vi "Configure.vi"(8 "error in (no error)":errorcluster, 10 "Msg in":T1, 11 "FakePressureController in":refnum<class "Tapedrive_ESP301.lvclass">) -> (0 "error out":errorcluster, 1 "new command":string, 2 "Msg out":T1, 3 "FakePressureController out":refnum<class "Tapedrive_ESP301.lvclass">)   [LabVIEW 2011, in "Tapedrive_ESP301.lvclass"]
uses:
  Tapedrive_ESP301.lvclass
  DriverMsg.ctl
  Tapedrive_ESP301.lvclass/Tapedrive_ESP301.ctl
  OnOffTypeDef.ctl
  Direction.ctl
  BaseDriver/BaseDriver.lvclass
  Newport ESP301.lvlib
panel:
  out "Command":string
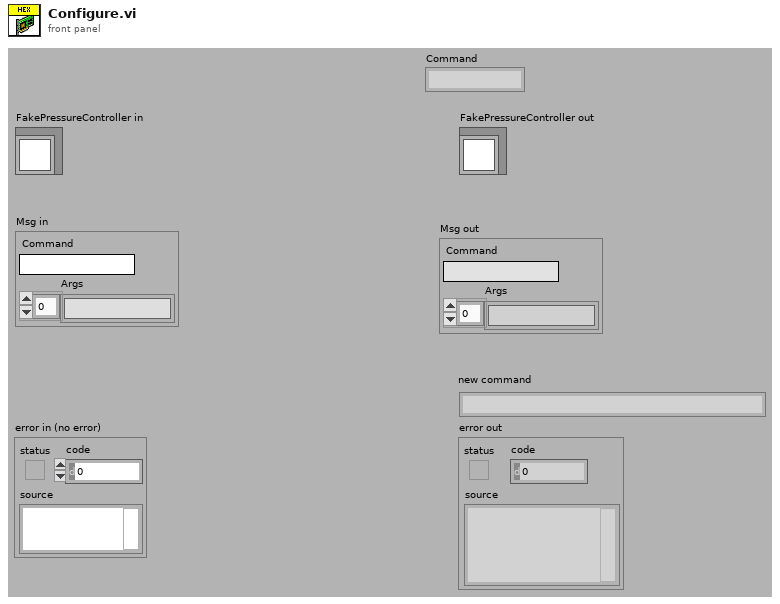
[diagram p1: front panel]
types:
  T1 = typedef "DriverMsg.ctl" = cluster{"Command":string, "Args":string[]}
  T2 = typedef "OnOffTypeDef.ctl" = enum16{"off", "on"}
  T3 = typedef "Direction.ctl" = enum16{"Forward", "Backward", "Undefined"}
  T4 = enum16{"Trapezoidal Mode", "S-curve Mode", "Jog Mode", "Slave to master's desired position (trajectory)", "Slave to master's actual position (feedback)", "Slave to master's actual velocity for jogging"}
  T5 = typedef "Tapedrive_ESP301.lvclass/settingsCluster_TapeDrive_TypDef.ctl" = cluster{"devport":string, "tapepos":cluster{"Value":dbl, "Min":dbl, "Max":dbl, "StepSize":dbl, "Tolerance":dbl, "ValueActual":dbl}, "status":enum16{"Not referenced", "Homing", "Moving", "Ready"}, "inmotion":T2, "forwardaxis":i16, "backwardaxis":i16, "encoderaxis":i16, "Velocity":cluster{"Axis 1":cluster{"Value":dbl, "Min":dbl, "Max":dbl, "StepSize":dbl, "Tolerance":dbl, "ValueActual":dbl}, "Axis 2":cluster{"Value":dbl, "Min":dbl, "Max":dbl, "StepSize":dbl, "Tolerance":dbl, "ValueActual":dbl}}, "Acceleration":cluster{"Axis 1":cluster{"Value":dbl, "Min":dbl, "Max":dbl, "StepSize":dbl, "Tolerance":dbl, "ValueActual":dbl}, "Axis 2":cluster{"Value":dbl, "Min":dbl, "Max":dbl, "StepSize":dbl, "Tolerance":dbl, "ValueActual":dbl}}, "Decceleration":cluster{"Axis 1":cluster{"Value":dbl, "Min":dbl, "Max":dbl, "StepSize":dbl, "Tolerance":dbl, "ValueActual":dbl}, "Axis 2":cluster{"Value":dbl, "Min":dbl, "Max":dbl, "StepSize":dbl, "Tolerance":dbl, "ValueActual":dbl}}, "MaxAcceleration":cluster{"Axis 1":cluster{"Value":dbl, "Min":dbl, "Max":dbl, "StepSize":dbl, "Tolerance":dbl, "ValueActual":dbl}, "Axis 2":cluster{"Value":dbl, "Min":dbl, "Max":dbl, "StepSize":dbl, "Tolerance":dbl, "ValueActual":dbl}}, "MaxVelocity":cluster{"Axis 1":cluster{"Value":dbl, "Min":dbl, "Max":dbl, "StepSize":dbl, "Tolerance":dbl, "ValueActual":dbl}, "Axis 2":cluster{"Value":dbl, "Min":dbl, "Max":dbl, "StepSize":dbl, "Tolerance":dbl, "ValueActual":dbl}}, "VelocityFFG":cluster{"Axis 1":cluster{"Value":dbl, "Min":dbl, "Max":dbl, "StepSize":dbl, "Tolerance":dbl, "ValueActual":dbl}, "Axis 2":cluster{"Value":dbl, "Min":dbl, "Max":dbl, "StepSize":dbl, "Tolerance":dbl, "ValueActual":dbl}}, "AccelerationFFG":cluster{"Axis 1":cluster{"Value":dbl, "Min":dbl, "Max":dbl, "StepSize":dbl, "Tolerance":dbl, "ValueActual":dbl}, "Axis 2":cluster{"Value":dbl, "Min":dbl, "Max":dbl, "StepSize":dbl, "Tolerance":dbl, "ValueActual":dbl}}, "DACoffset":cluster{"Axis 1":cluster{"Value":dbl, "Min":dbl, "Max":dbl, "StepSize":dbl, "Tolerance":dbl, "ValueActual":dbl}, "Axis 2":cluster{"Value":dbl, "Min":dbl, "Max":dbl, "StepSize":dbl, "Tolerance":dbl, "ValueActual":dbl}}, "Power":cluster{"Axis 1":T2, "Axis 2":T2}, "ReductionRatio":cluster{"Value":dbl, "Min":dbl, "Max":dbl, "StepSize":dbl, "Tolerance":dbl, "ValueActual":dbl}, "Direction":T3, "Tension":T2, "TensionVelocity":cluster{"Axis 1":cluster{"Value":dbl, "Min":dbl, "Max":dbl, "StepSize":dbl, "Tolerance":dbl, "ValueActual":dbl}, "Axis 2":cluster{"Value":dbl, "Min":dbl, "Max":dbl, "StepSize":dbl, "Tolerance":dbl, "ValueActual":dbl}}, "TensionAcceleration":cluster{"Axis 1":cluster{"Value":dbl, "Min":dbl, "Max":dbl, "StepSize":dbl, "Tolerance":dbl, "ValueActual":dbl}, "Axis 2":cluster{"Value":dbl, "Min":dbl, "Max":dbl, "StepSize":dbl, "Tolerance":dbl, "ValueActual":dbl}}, "TensionDecceleration":cluster{"Axis 1":cluster{"Value":dbl, "Min":dbl, "Max":dbl, "StepSize":dbl, "Tolerance":dbl, "ValueActual":dbl}, "Axis 2":cluster{"Value":dbl, "Min":dbl, "Max":dbl, "StepSize":dbl, "Tolerance":dbl, "ValueActual":dbl}}, "MoveVelocity":cluster{"Axis 1":cluster{"Value":dbl, "Min":dbl, "Max":dbl, "StepSize":dbl, "Tolerance":dbl, "ValueActual":dbl}, "Axis 2":cluster{"Value":dbl, "Min":dbl, "Max":dbl, "StepSize":dbl, "Tolerance":dbl, "ValueActual":dbl}}, "MoveAcceleration":cluster{"Axis 1":cluster{"Value":dbl, "Min":dbl, "Max":dbl, "StepSize":dbl, "Tolerance":dbl, "ValueActual":dbl}, "Axis 2":cluster{"Value":dbl, "Min":dbl, "Max":dbl, "StepSize":dbl, "Tolerance":dbl, "ValueActual":dbl}}, "MoveDecceleration":cluster{"Axis 1":cluster{"Value":dbl, "Min":dbl, "Max":dbl, "StepSize":dbl, "Tolerance":dbl, "ValueActual":dbl}, "Axis 2":cluster{"Value":dbl, "Min":dbl, "Max":dbl, "StepSize":dbl, "Tolerance":dbl, "ValueActual":dbl}}, "MaxStepsize":cluster{"Value":dbl, "Min":dbl, "Max":dbl, "StepSize":dbl, "Tolerance":dbl, "ValueActual":dbl}, "Stepsize":cluster{"Value":dbl, "Min":dbl, "Max":dbl, "StepSize":dbl, "Tolerance":dbl, "ValueActual":dbl}, "GoStep":T2, "StopWait":T2, "stepnum":cluster{"Value":dbl, "Min":dbl, "Max":dbl, "StepSize":dbl, "Tolerance":dbl, "ValueActual":dbl}, "MoveIfScan":T2, "HomeEncoder":T2, "Timeout":cluster{"Value":dbl, "Min":dbl, "Max":dbl, "StepSize":dbl, "Tolerance":dbl, "ValueActual":dbl}, "TapeRelax":cluster{"Value":dbl, "Min":dbl, "Max":dbl, "StepSize":dbl, "Tolerance":dbl, "ValueActual":dbl}}
  T6 = cluster{"Axis 1":cluster{"Value":dbl, "Min":dbl, "Max":dbl, "StepSize":dbl, "Tolerance":dbl, "ValueActual":dbl}, "Axis 2":cluster{"Value":dbl, "Min":dbl, "Max":dbl, "StepSize":dbl, "Tolerance":dbl, "ValueActual":dbl}}
  T7 = cluster{"Axis 1":cluster{"Value":dbl, "Min":dbl, "Max":dbl, "StepSize":dbl, "Tolerance":dbl, "ValueActual":dbl}, "Axis 2":cluster{"Value":dbl, "Min":dbl, "Max":dbl, "StepSize":dbl, "Tolerance":dbl, "ValueActual":dbl}}[]
  T8 = enum16{"Not referenced", "Homing", "Moving", "Ready"}
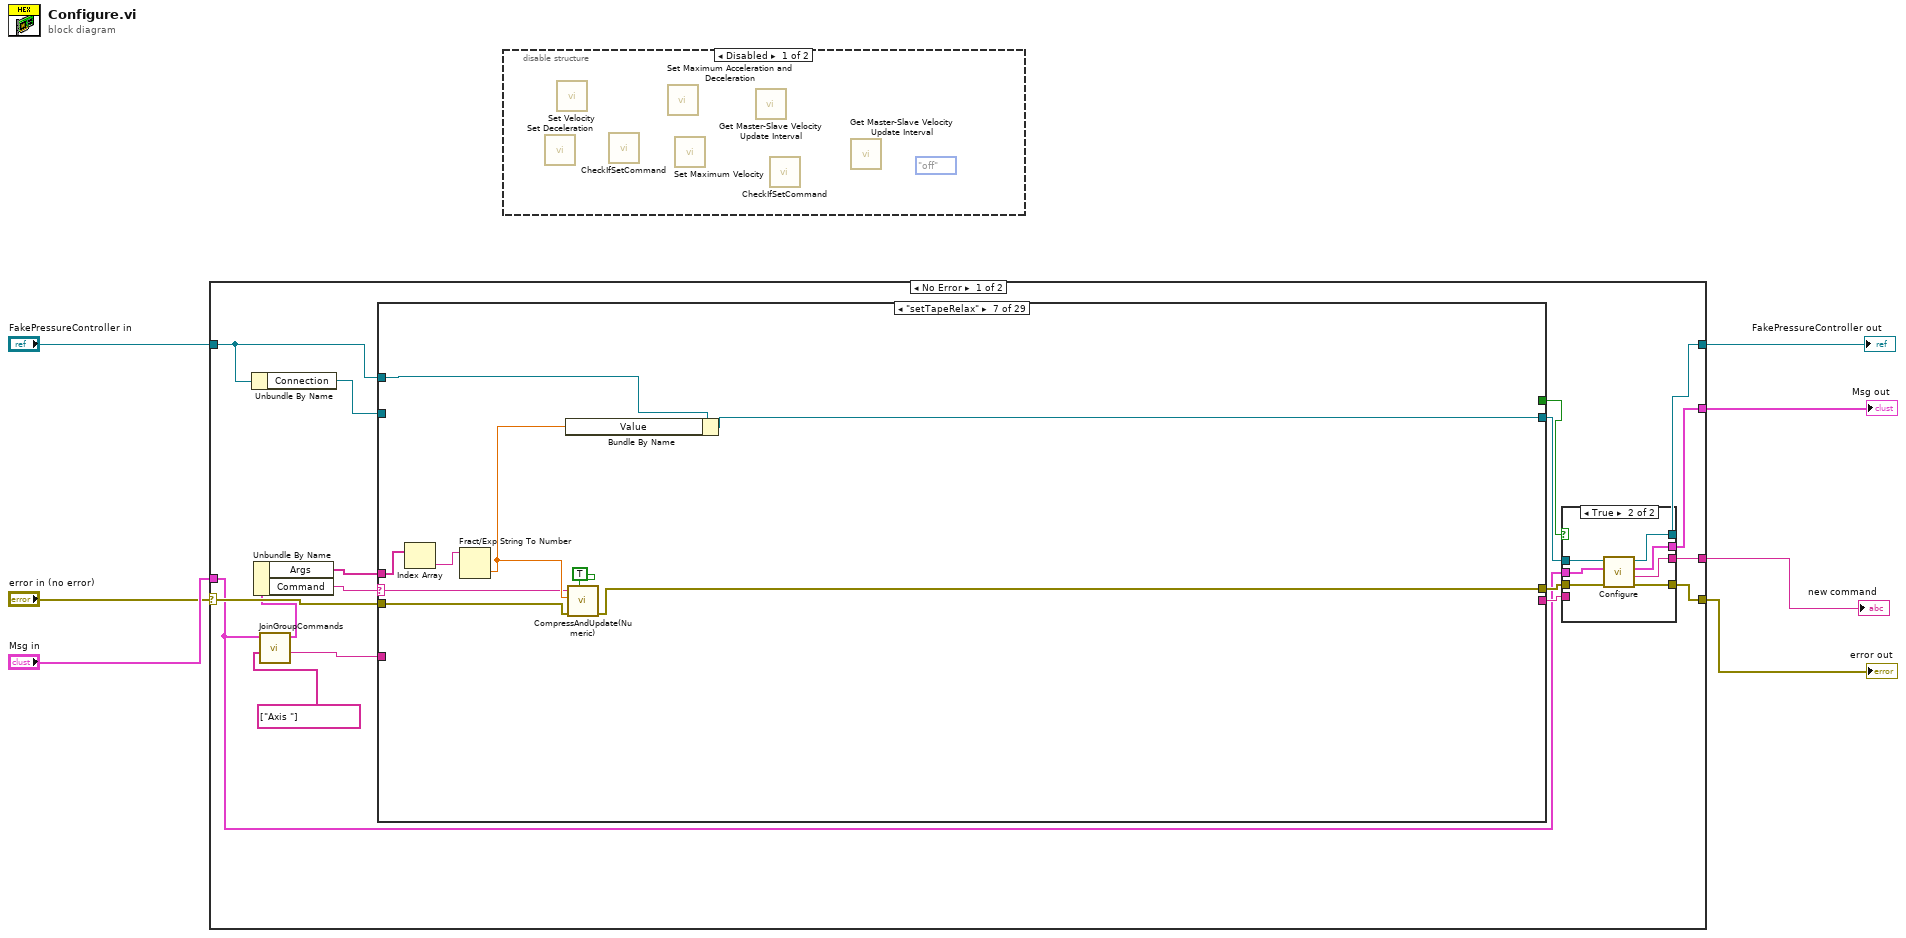
[diagram p0: block diagram]
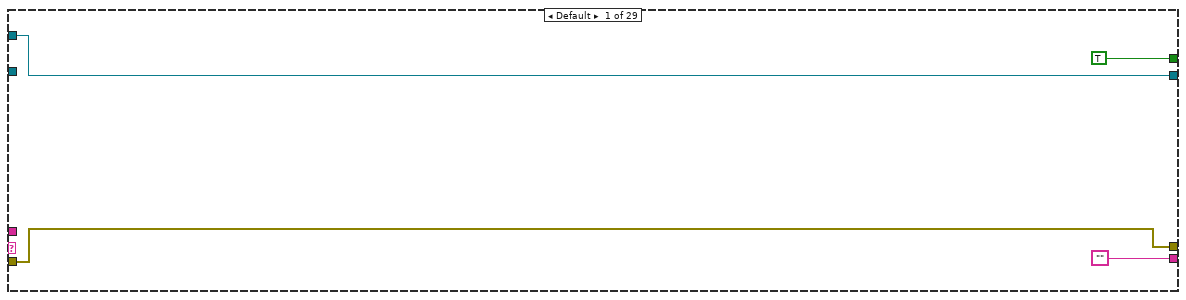
[diagram p4: hidden frame]
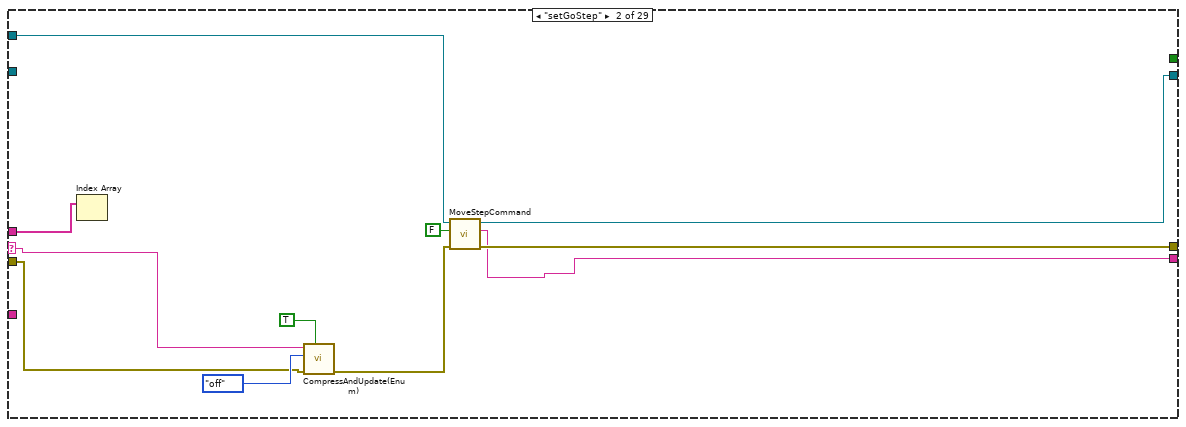
[diagram p5: hidden frame]
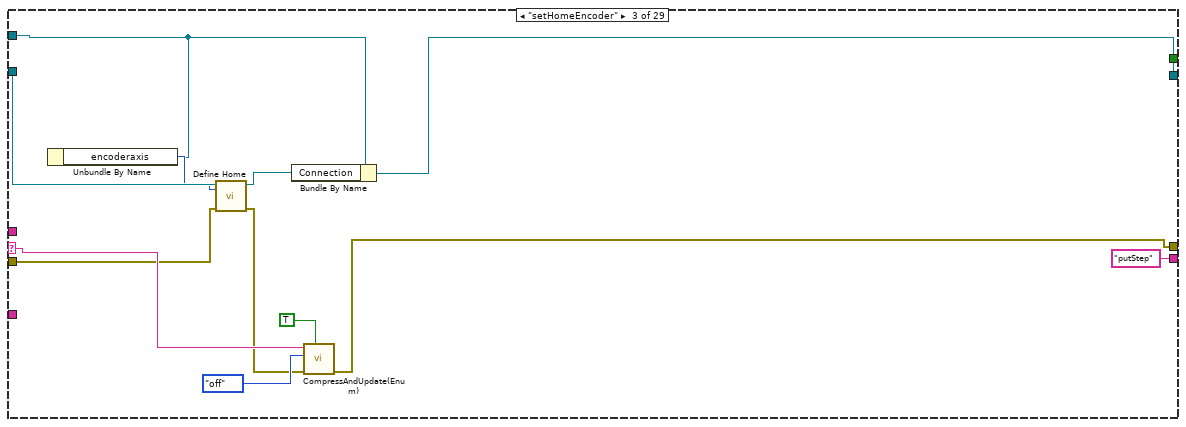
[diagram p6: hidden frame]
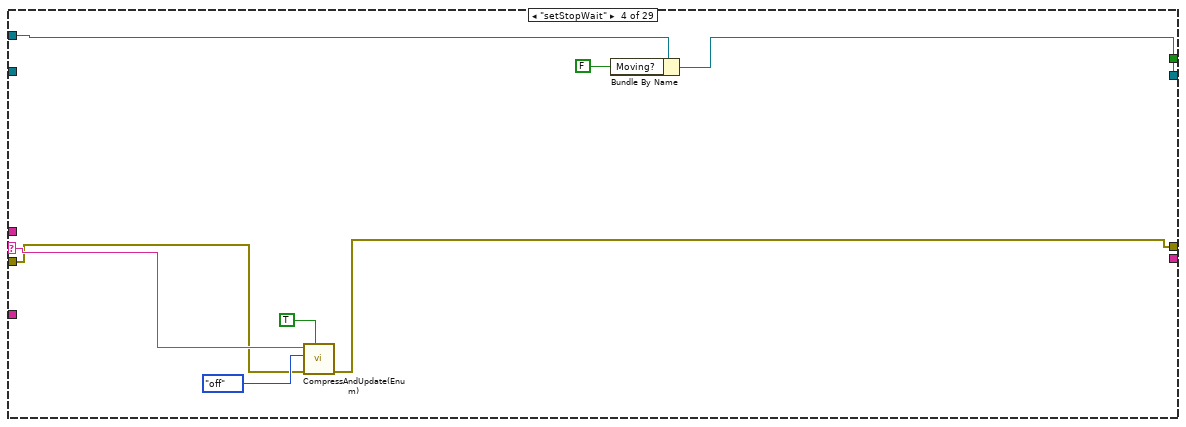
[diagram p7: hidden frame]
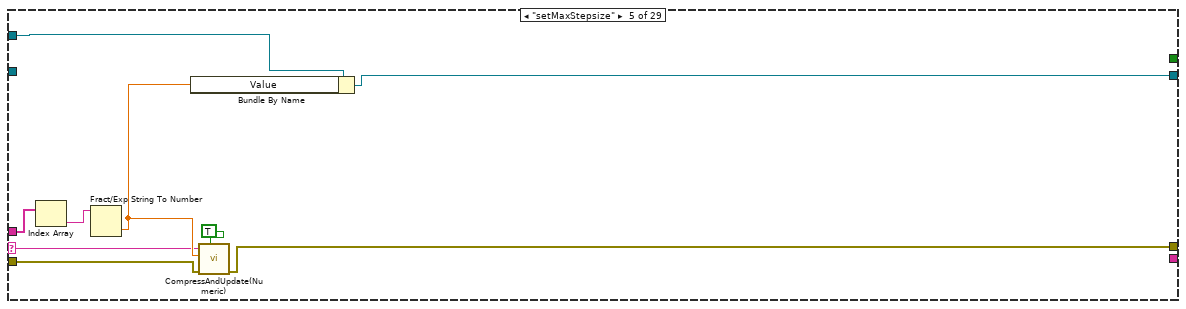
[diagram p8: hidden frame]
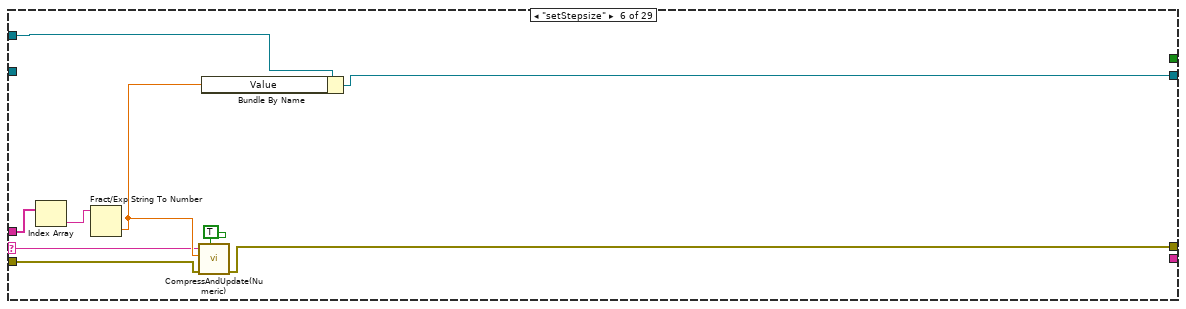
[diagram p9: hidden frame]
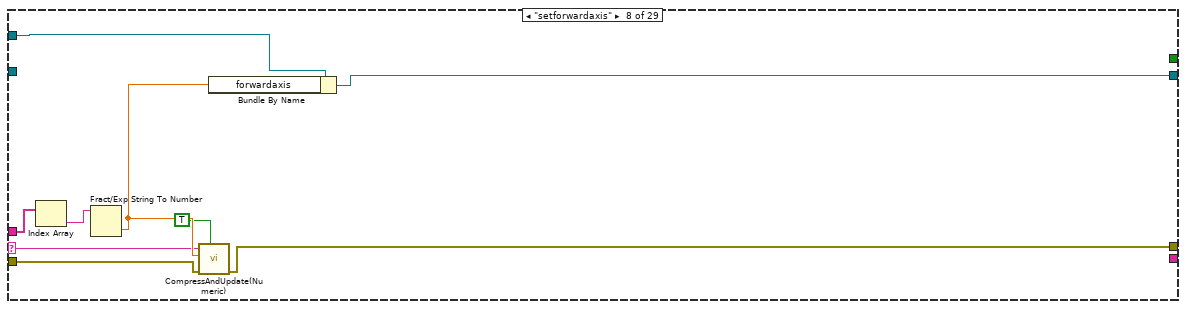
[diagram p10: hidden frame]
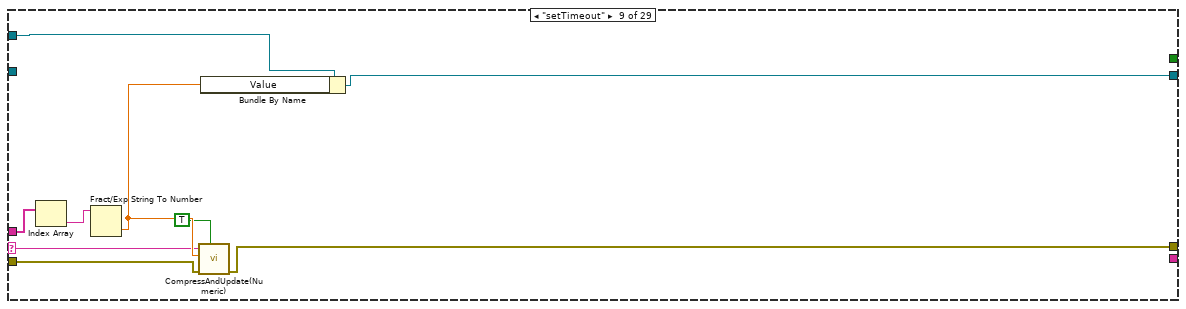
[diagram p11: hidden frame]
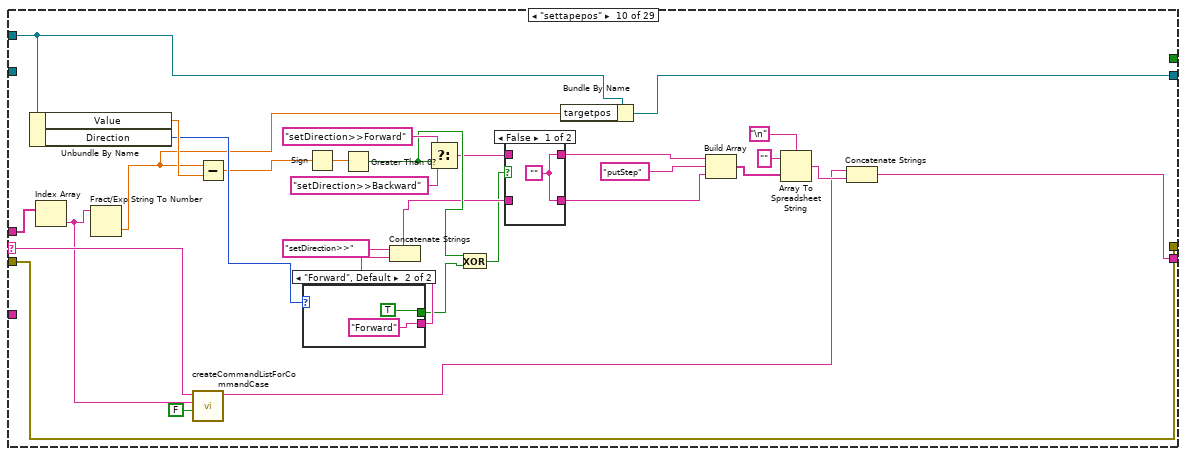
[diagram p12: hidden frame]
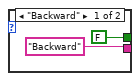
[diagram p14: hidden frame]
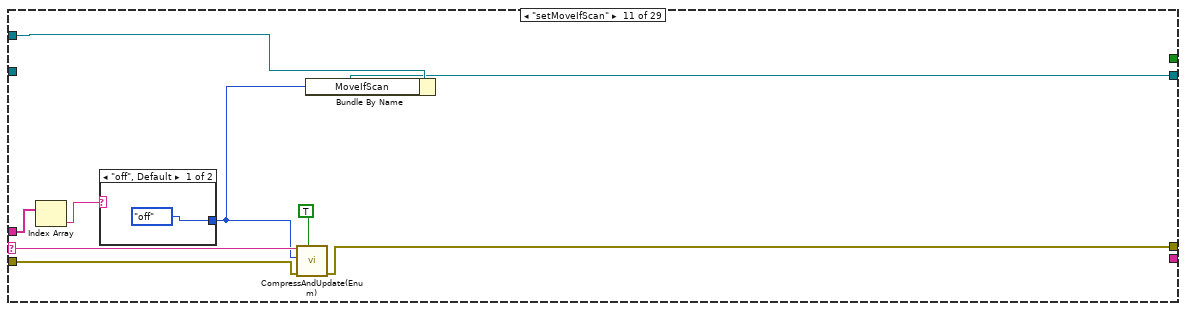
[diagram p15: hidden frame]
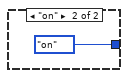
[diagram p16: hidden frame]
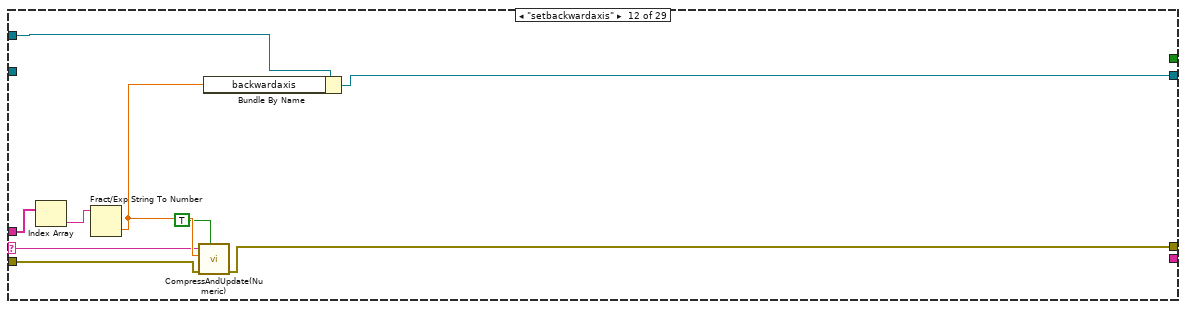
[diagram p17: hidden frame]
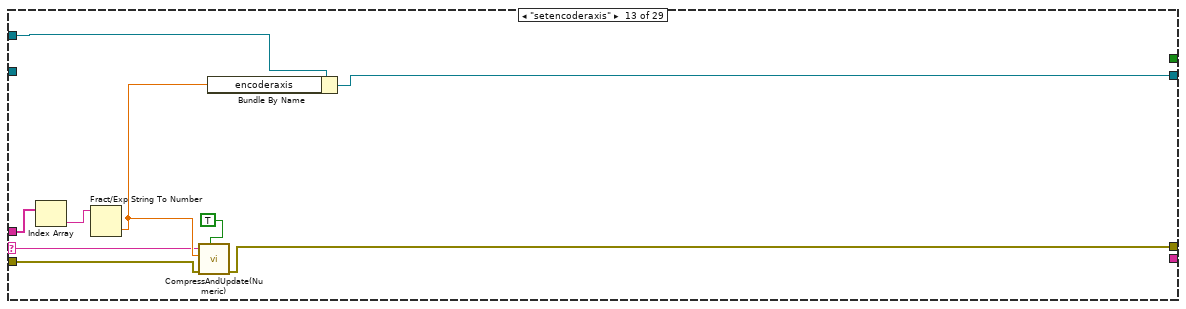
[diagram p18: hidden frame]
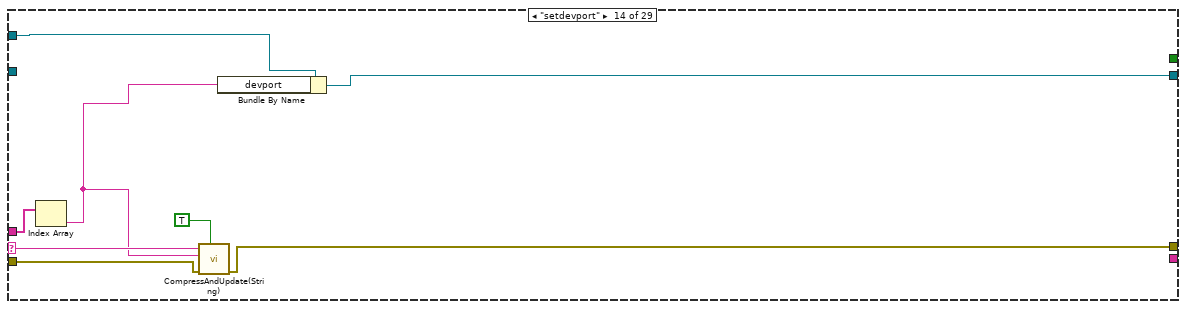
[diagram p19: hidden frame]
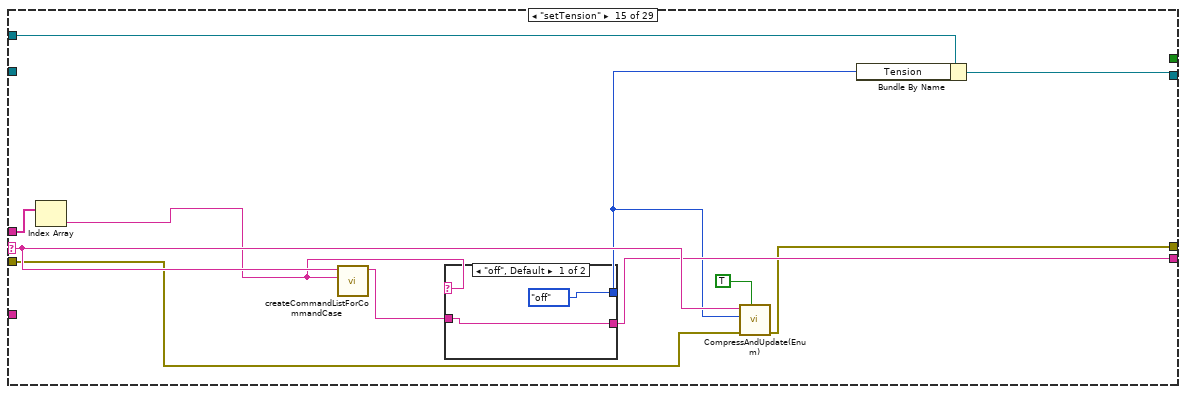
[diagram p20: hidden frame]
diagram:
  n1 = case shown="No Error" "error in (no error)" {
    selector: "error in (no error)" -> [w16 w794]
    tunnel: "FakePressureController in" -> [w13 w792]
    tunnel: [w23 w792] -> w3
    tunnel: [w21 w794] -> w4
    tunnel: "Msg in" -> [w8 w793]
    tunnel: [w19 w793] -> w2
    tunnel: [w17 _] -> w1
    frame No Error {
      n2 = Unbundle By Name(w13) -> ("Connection"=w12:refnum<visa-resource-name>)
      n3 = call "JoinGroupCommands.vi"("Seperator"=string[] ["Axis "], "Msg in"=w8) -> ("Seperator out"=w9:string, "Msg out"=w11:T1)  [unwired: 7 in, 1 out]
      n4 = Unbundle By Name(w11) -> ("Args"=w15:string[], "Command"=w14:string)
      n5 = case shown="\"setTapeRelax\"" w14 {
        selector: w14 -> [_ w42 w61 w70 w74 w83 w92 w101 w110 w134 w158 w167 w176 w186 w196 w227 w341 w365 w390 w497 w527 _ _ _ _ w653 _ _ _]
        tunnel: w16 -> [w38 w48 w55 w67 w73 w82 w91 w100 w109 w144 w157 w166 w175 w185 w192 w240 w350 w361 w392 w486 w510 w546 w574 w581 w594 w665 w680 w743 w764]
        tunnel: w15 -> [_ w41 _ _ w77 w86 w95 w104 w113 w145 w159 w170 w179 w187 w198 w239 w349 w372 w405 w483 w517 w555 _ w580 _ w664 _ w748 w762]
        tunnel: w13 -> [w39 w46 w53 w65 w79 w88 w97 w106 w115 w139 w161 w172 w181 w189 w200 w232 w343 w368 w398 w490 w520 w545 w573 w582 w589 w661 w675 w739 w766]
        tunnel: [w39 w45 w52 w64 w78 w87 w96 w105 w114 w138 w160 w171 w180 w188 w199 w229 w342 w366 w394 w488 w518 w544 w571 w582 w586 w660 w672 w738 w767] -> w24
        tunnel: ["" ("Complete") w40 "putStep" ("spreadsheet string") _ _ _ _ _ _ w129 _ _ _ _ w193 w214 w325 w362 w399 w491 w521 _ _ _ w595 _ w681 w735 _] -> w18
        tunnel: [w38 w47 w58 w66 w72 w81 w90 w99 w108 w144 w156 w165 w174 w184 w191 w211 w328 w360 w388 w471 w506 w532 w570 w581 w588 w654 w674 w742 w763] -> w22
        tunnel: [TRUE _ _ _ _ _ _ _ _ _ _ _ _ _ _ _ _ _ _ _ _ _ _ _ _ _ _ _ _] -> w20
        tunnel: w12 -> [_ _ w57 _ _ _ _ _ _ _ _ _ _ _ _ w241 w351 _ w391 w487 w511 _ w577 _ w592 w669 w678 w745 w765]
        tunnel: w9 -> [_ _ _ _ _ _ _ _ _ _ _ _ _ _ _ w237 w347 _ w403 w495 w525 _ _ _ _ _ _ _ _]
        frame Default {
        }
        frame "setGoStep" {
          n6 = Index Array(array=w41) -> ()  [unwired: 1 in, 1 out]
          n7 = call "CompressAndUpdate(Enum).vi"("force CVT update (false)"=TRUE, "error in"=w48, "enum variant"=OnOffTypeDef."off" ("inmotion"), "command or variable name"=w42) -> ("error out"=w43:errorcluster)  [unwired: 7 in]
          n8 = call "MoveStepCommand.vi"("error in (no error)"=w43, "MultiCVT"=FALSE, "Tapedrive_ESP301 in"=w46) -> ("error out"=w47:errorcluster, "String"=w40:string, "Tapedrive_ESP301.lvclass"=w45:refnum<class "Tapedrive_ESP301.lvclass">)  [unwired: 6 in]
        }
        frame "setHomeEncoder" {
          n9 = Unbundle By Name(w53) -> ("encoderaxis"=w56:i16)
          n10 = call "Define Home.vi"("error in (no error)"=w55, "Axis (1)"=w56, "VISA resource name"=w57) -> ("error out"=w54:errorcluster, "VISA resource name out"=w51:refnum<visa-resource-name>)  [unwired: 3 in]
          n11 = Bundle By Name(cluster=w53, "Connection"=w51) -> (w52:refnum<class "Tapedrive_ESP301.lvclass">)
          n12 = call "CompressAndUpdate(Enum).vi"("force CVT update (false)"=TRUE, "error in"=w54, "enum variant"=OnOffTypeDef."off" ("inmotion"), "command or variable name"=w61) -> ("error out"=w58:errorcluster)  [unwired: 7 in]
        }
        frame "setStopWait" {
          n13 = call "CompressAndUpdate(Enum).vi"("force CVT update (false)"=TRUE, "error in"=w67, "enum variant"=OnOffTypeDef."off" ("inmotion"), "command or variable name"=w70) -> ("error out"=w66:errorcluster)  [unwired: 7 in]
          n14 = Bundle By Name(cluster=w65, "Moving?"=FALSE ("Wait for Step")) -> (w64:refnum<class "Tapedrive_ESP301.lvclass">)
        }
        frame "setMaxStepsize" {
          n15 = Index Array(array=w77) -> (element=w76:string)  [unwired: 1 in]
          n16 = Fract/Exp String To Number(string=w76) -> (number=w75:dbl)  [unwired: 3 in, 1 out]
          n17 = Bundle By Name(cluster=w79, "Value"=w75) -> (w78:refnum<class "Tapedrive_ESP301.lvclass">)
          n18 = call "CompressAndUpdate(Numeric).vi"("force CVT update (false)"=TRUE, "error in"=w73, "Numeric"=w75, "command or variable name"=w74) -> ("error out"=w72:errorcluster)  [unwired: 7 in]
        }
        frame "setStepsize" {
          n19 = Index Array(array=w86) -> (element=w85:string)  [unwired: 1 in]
          n20 = Fract/Exp String To Number(string=w85) -> (number=w84:dbl)  [unwired: 3 in, 1 out]
          n21 = call "CompressAndUpdate(Numeric).vi"("force CVT update (false)"=TRUE, "error in"=w82, "Numeric"=w84, "command or variable name"=w83) -> ("error out"=w81:errorcluster)  [unwired: 7 in]
          n22 = Bundle By Name(cluster=w88, "Value"=w84) -> (w87:refnum<class "Tapedrive_ESP301.lvclass">)
        }
        frame "setTapeRelax" {
          n23 = Index Array(array=w95) -> (element=w94:string)  [unwired: 1 in]
          n24 = Fract/Exp String To Number(string=w94) -> (number=w93:dbl)  [unwired: 3 in, 1 out]
          n25 = Bundle By Name(cluster=w97, "Value"=w93) -> (w96:refnum<class "Tapedrive_ESP301.lvclass">)
          n26 = call "CompressAndUpdate(Numeric).vi"("force CVT update (false)"=TRUE, "error in"=w91, "Numeric"=w93, "command or variable name"=w92) -> ("error out"=w90:errorcluster)  [unwired: 7 in]
        }
        frame "setforwardaxis" {
          n27 = Index Array(array=w104) -> (element=w103:string)  [unwired: 1 in]
          n28 = Fract/Exp String To Number(string=w103) -> (number=w102:dbl)  [unwired: 3 in, 1 out]
          n29 = call "CompressAndUpdate(Numeric).vi"("force CVT update (false)"=TRUE, "error in"=w100, "Numeric"=w102, "command or variable name"=w101) -> ("error out"=w99:errorcluster)  [unwired: 7 in]
          n30 = Bundle By Name(cluster=w106, "forwardaxis"=w102) -> (w105:refnum<class "Tapedrive_ESP301.lvclass">)
        }
        frame "setTimeout" {
          n31 = Index Array(array=w113) -> (element=w112:string)  [unwired: 1 in]
          n32 = Fract/Exp String To Number(string=w112) -> (number=w111:dbl)  [unwired: 3 in, 1 out]
          n33 = call "CompressAndUpdate(Numeric).vi"("force CVT update (false)"=TRUE, "error in"=w109, "Numeric"=w111, "command or variable name"=w110) -> ("error out"=w108:errorcluster)  [unwired: 7 in]
          n34 = Bundle By Name(cluster=w115, "Value"=w111) -> (w114:refnum<class "Tapedrive_ESP301.lvclass">)
        }
        frame "settapepos" {
          n35 = Unbundle By Name(w139) -> ("Value"=w143:dbl, "Direction"=w126:T3)
          n36 = Index Array(array=w145) -> (element=w133:string)  [unwired: 1 in]
          n37 = Fract/Exp String To Number(string=w133) -> (number=w117:dbl)  [unwired: 3 in, 1 out]
          n38 = call "createCommandListForCommandCase.vi"("immediate Check (only once)"=FALSE, "setvalue"=w133, "command"=w134) -> ("new commands"=w130:string)  [unwired: 8 in]
          n39 = Subtract(x=w117, y=w143) -> (x-y=w116:dbl)
          n40 = case shown="\"Forward\", Default" w126 {
            tunnel: ["Backward" "Forward"] -> w125
            tunnel: [FALSE TRUE] -> w123
            frame "Backward" {
            }
            frame "Forward", Default {
            }
          }
          n41 = Sign(1:w116) -> (0:w142:dbl)
          n42 = Greater Than 0?(x=w142) -> (x > 0?=w124:bool)
          n43 = Concatenate Strings("setDirection>>", w125) -> (w120:string)
          n44 = Select(t="setDirection>>Forward", s=w124, f="setDirection>>Backward") -> (s? t:f=w122:string)
          n45 = Exclusive Or(1:w123, 2:w124) -> (0:w118:bool)
          n46 = case shown="False" w118 {
            tunnel: w122 -> [_ w148]
            tunnel: [w146 w148] -> w121
            tunnel: w120 -> [_ w147]
            tunnel: [w146 w147] -> w119
            frame False {
              w146 = ""
            }
            frame True {
            }
          }
          n47 = Bundle By Name(cluster=w139, "targetpos"=w117) -> (w138:refnum<class "Tapedrive_ESP301.lvclass">)
          n48 = Build Array(w121, "putStep", w119) -> (w137:string[])
          n49 = Array To Spreadsheet String(delimiter (Tab)="\n", array=w137, 3:"" ("format string")) -> (spreadsheet string=w131:string)
          n50 = Concatenate Strings(w130, w131) -> (w129:string)
        }
        frame "setMoveIfScan" {
          n51 = Index Array(array=w159) -> (element=w154:string)  [unwired: 1 in]
          n52 = case shown="\"off\", Default" w154 {
            tunnel: [OnOffTypeDef."off" ("inmotion") OnOffTypeDef."on" ("inmotion")] -> w153
            frame "off", Default {
            }
            frame "on" {
            }
          }
          n53 = call "CompressAndUpdate(Enum).vi"("force CVT update (false)"=TRUE, "error in"=w157, "enum variant"=w153, "command or variable name"=w158) -> ("error out"=w156:errorcluster)  [unwired: 7 in]
          n54 = Bundle By Name(cluster=w161, "MoveIfScan"=w153) -> (w160:refnum<class "Tapedrive_ESP301.lvclass">)
        }
        frame "setbackwardaxis" {
          n55 = Index Array(array=w170) -> (element=w169:string)  [unwired: 1 in]
          n56 = Fract/Exp String To Number(string=w169) -> (number=w168:dbl)  [unwired: 3 in, 1 out]
          n57 = call "CompressAndUpdate(Numeric).vi"("force CVT update (false)"=TRUE, "error in"=w166, "Numeric"=w168, "command or variable name"=w167) -> ("error out"=w165:errorcluster)  [unwired: 7 in]
          n58 = Bundle By Name(cluster=w172, "backwardaxis"=w168) -> (w171:refnum<class "Tapedrive_ESP301.lvclass">)
        }
        frame "setencoderaxis" {
          n59 = Index Array(array=w179) -> (element=w178:string)  [unwired: 1 in]
          n60 = Fract/Exp String To Number(string=w178) -> (number=w177:dbl)  [unwired: 3 in, 1 out]
          n61 = call "CompressAndUpdate(Numeric).vi"("force CVT update (false)"=TRUE, "error in"=w175, "Numeric"=w177, "command or variable name"=w176) -> ("error out"=w174:errorcluster)  [unwired: 7 in]
          n62 = Bundle By Name(cluster=w181, "encoderaxis"=w177) -> (w180:refnum<class "Tapedrive_ESP301.lvclass">)
        }
        frame "setdevport" {
          n63 = Index Array(array=w187) -> (element=w183:string)  [unwired: 1 in]
          n64 = call "CompressAndUpdate(String).vi"("force CVT update (false)"=TRUE, "error in"=w185, "String"=w183, "command or variable name"=w186) -> ("error out"=w184:errorcluster)  [unwired: 7 in]
          n65 = Bundle By Name(cluster=w189, "devport"=w183) -> (w188:refnum<class "Tapedrive_ESP301.lvclass">)
        }
        frame "setTension" {
          n66 = Index Array(array=w198) -> (element=w195:string)  [unwired: 1 in]
          n67 = call "createCommandListForCommandCase.vi"("setvalue"=w195, "command"=w196) -> ("new commands"=w194:string)  [unwired: 9 in]
          n68 = case shown="\"off\", Default" w195 {
            tunnel: w194 -> [w201 w206]
            tunnel: [w201 w204] -> w193
            tunnel: [OnOffTypeDef."off" ("Tension") OnOffTypeDef."on" ("Tension")] -> w190
            frame "off", Default {
            }
            frame "on" {
              n69 = Concatenate Strings(w206, "putTension" ("string")) -> (w204:string)
            }
          }
          n70 = call "CompressAndUpdate(Enum).vi"("force CVT update (false)"=TRUE, "error in"=w192, "enum variant"=w190, "command or variable name"=w196) -> ("error out"=w191:errorcluster)  [unwired: 7 in]
          n71 = Bundle By Name(cluster=w200, "Tension"=w190) -> (w199:refnum<class "Tapedrive_ESP301.lvclass">)
        }
        frame "setAcceleration", "setAccelerationFFG", "setDecceleration", "setMaxAcceleration", "setMaxVelocity", "setVelocity", "setVelocityFFG" {
          n72 = call "reBuildJoindCommand.vi"("number of group elements (0)"=1, "Args"=w239, "Command 2"=w227) -> ("Arg"=w234:string, "Command"=w225:string)
          n73 = Unbundle By Name(w232) -> ("Settings"=w210:T5, "forwardaxis"=w221:i16, "backwardaxis"=w220:i16)
          n74 = call "CheckIfSetCommand.vi"("Command"=w227) -> ("variable"=w226:string)  [unwired: 2 out]
          n75 = call "getSeperator.vi"("Channel Seperator (\"\")"=w237, "Command"=w225) -> ("Channel"=w236:string)  [unwired: 8 in, 1 out]
          n76 = Decimal String To Number(string=w236) -> (number=w219:i32)  [unwired: 2 in, 1 out]
          n77 = Build Array(w221, w220) -> (w217:i16[])
          n78 = Decrement(x=w219) -> (x-1=w218:i32)
          n79 = Fract/Exp String To Number(string=w234) -> (number=w235:dbl)  [unwired: 3 in, 1 out]
          n80 = Index Array(array=w217, index=w218) -> (element=w216:i16)
          n81 = case shown="\"Velocity\", Default" w226 {
            tunnel: w241 -> [w251 w261 w271 w281 w291 w301 w311]
            tunnel: w240 -> [w250 w260 w269 w279 w284 w299 w307]
            tunnel: w216 -> [w245 w257 w263 w274 w289 w295 w303]
            tunnel: w235 -> [w249 w256 w270 w280 w282 w300 w306]
            tunnel: [w243 w255 w264 w273 w286 w293 w304] -> w223
            tunnel: [w244 w254 w265 w275 w288 w296 w308] -> w224
            tunnel: [w246 w253 w266 w276 w287 w297 w309] -> w228
            tunnel: 100 -> [w242 w252 w262 w272 w283 w292 w302]
            frame "Velocity", Default {
              n82 = call "Set Velocity.vi"("error in (no error)"=w250, "Velocity (units/s)"=w249, "Axis (1)"=w245, "VISA resource name"=w251) -> ("error out"=w247:errorcluster, "VISA resource name out"=w248:refnum<visa-resource-name>)  [unwired: 2 in]
              n83 = call "Get Velocity.vi"("error in (no error)"=w247, "Wait before read (0ms)"=w242, "Axis (1)"=w245, "VISA resource name"=w248) -> ("error out"=w243:errorcluster, "Velocity (units/s)"=w244:dbl, "VISA resource name out"=w246:refnum<visa-resource-name>)  [unwired: 1 in]
            }
            frame "Acceleration" {
              n84 = call "Set Acceleration.vi"("error in (no error)"=w260, "Acceleration (0 units/s²)"=w256, "Axis (1)"=w257, "VISA resource name"=w261) -> ("error out"=w259:errorcluster, "VISA resource name out"=w258:refnum<visa-resource-name>)  [unwired: 2 in]
              n85 = call "Get Acceleration.vi"("error in (no error)"=w259, "Wait before read (0ms)"=w252, "Axis (1)"=w257, "VISA resource name"=w258) -> ("error out"=w255:errorcluster, "Acceleration (units/s²)"=w254:dbl, "VISA resource name out"=w253:refnum<visa-resource-name>)  [unwired: 1 in]
            }
            frame "Decceleration" {
              n86 = call "Set Deceleration.vi"("error in (no error)"=w269, "Deceleration (0 units/s²)"=w270, "Axis (1)"=w263, "VISA resource name"=w271) -> ("error out"=w268:errorcluster, "VISA resource name out"=w267:refnum<visa-resource-name>)  [unwired: 2 in]
              n87 = call "Get Deceleration.vi"("error in (no error)"=w268, "Wait before read (0ms)"=w262, "Axis (1)"=w263, "VISA resource name"=w267) -> ("error out"=w264:errorcluster, "Deceleration (units/s²)"=w265:dbl, "VISA resource name out"=w266:refnum<visa-resource-name>)  [unwired: 1 in]
            }
            frame "MaxVelocity" {
              n88 = call "Set Maximum Velocity.vi"("error in (no error)"=w279, "Maximum Velocity (0 units/s)"=w280, "Axis (1)"=w274, "VISA resource name"=w281) -> ("error out"=w278:errorcluster, "VISA resource name out"=w277:refnum<visa-resource-name>)  [unwired: 2 in]
              n89 = call "Get Maximum Velocity.vi"("error in (no error)"=w278, "Wait before read (0ms)"=w272, "Axis (1)"=w274, "VISA resource name"=w277) -> ("error out"=w273:errorcluster, "Maximum Velocity (units/s)"=w275:dbl, "VISA resource name out"=w276:refnum<visa-resource-name>)  [unwired: 1 in]
            }
            frame "MaxAcceleration" {
              n90 = call "Set Maximum Acceleration and Deceleration.vi"("error in (no error)"=w284, "Acceleration (0 units/s²)"=w282, "Axis (1)"=w289, "VISA resource name"=w291) -> ("error out"=w285:errorcluster, "VISA resource name out"=w290:refnum<visa-resource-name>)  [unwired: 2 in]
              n91 = call "Get Maximum Acceleration and Deceleration.vi"("error in (no error)"=w285, "Wait before read (0ms)"=w283, "Axis (1)"=w289, "VISA resource name"=w290) -> ("error out"=w286:errorcluster, "Acceleration (units/s²)"=w288:dbl, "VISA resource name out"=w287:refnum<visa-resource-name>)  [unwired: 1 in]
            }
            frame "VelocityFFG" {
              n92 = call "Set Velocity Feed-Forward Gain.vi"("error in (no error)"=w299, "Velocity feed-forward gain factor (0)"=w300, "Axis (1)"=w295, "VISA resource name"=w301) -> ("error out"=w294:errorcluster, "VISA resource name out"=w298:refnum<visa-resource-name>)  [unwired: 2 in]
              n93 = call "Get Velocity Feed-Forward Gain.vi"("error in (no error)"=w294, "Wait before read (0ms)"=w292, "Axis (1)"=w295, "VISA resource name"=w298) -> ("error out"=w293:errorcluster, "Gain"=w296:dbl, "VISA resource name out"=w297:refnum<visa-resource-name>)  [unwired: 1 in]
            }
            frame "AccelerationFFG" {
              n94 = call "Set Acceleration Feed-Forward Gain.vi"("error in (no error)"=w307, "Acceleration feed-forward gain factor (0)"=w306, "Axis (1)"=w303, "VISA resource name"=w311) -> ("error out"=w305:errorcluster, "VISA resource name out"=w310:refnum<visa-resource-name>)  [unwired: 2 in]
              n95 = call "Get Acceleration Feed-Forward Gain.vi"("error in (no error)"=w305, "Wait before read (0ms)"=w302, "Axis (1)"=w303, "VISA resource name"=w310) -> ("error out"=w304:errorcluster, "Gain"=w308:dbl, "VISA resource name out"=w309:refnum<visa-resource-name>)  [unwired: 1 in]
            }
          }
          n96 = call "createCommandListForCommandCase.vi"("immediate Check (only once)"=TRUE, "setvalue"=w234, "command"=w225) -> ("new commands"=w214:string)  [unwired: 8 in]
          n97 = call "CheckIfSetCommand.vi"("Command"=w225) -> ("variable"=w209:string)  [unwired: 2 out]
          n98 = Concatenate Strings(w209, ".Value" ("string")) -> (w207:string)
          n99 = call "CompressAndUpdate(Numeric).vi"("force CVT update (false)"=TRUE, "error in"=w223, "Numeric"=w224, "command or variable name"=w225) -> ("error out"=w213:errorcluster)  [unwired: 7 in]
          n100 = call "Set Cluster Element by Name__ogtk_TS.vi"("error in (no error)"=w213, "Element Name (\"\": New Element Data Name)"=w207, "New Element Value"=w224, "Cluster"=w210) -> ("error out"=w212:errorcluster, "VCluster out"=w231:variant)  [unwired: 5 in, 1 out]
          n101 = Variant To Data(error in=w212, type=w210, Variant=w231) -> (data=w230:T5, error out=w211:errorcluster)
          n102 = Bundle By Name(cluster=w232, "Settings"=w230, "Connection"=w228) -> (w229:refnum<class "Tapedrive_ESP301.lvclass">)
        }
        frame "setDACoffset" {
          n103 = call "reBuildJoindCommand.vi"("number of group elements (0)"=1, "Args"=w349, "Command 2"=w341) -> ("Arg"=w345:string, "Command"=w312:string)
          n104 = Unbundle By Name(w343) -> ("Settings"=w327:T5, "forwardaxis"=w340:i16, "backwardaxis"=w339:i16)
          n105 = call "getSeperator.vi"("Channel Seperator (\"\")"=w347, "Command"=w312) -> ("Channel"=w324:string)  [unwired: 8 in, 1 out]
          n106 = call "CheckIfSetCommand.vi"("Command"=w312) -> ("variable"=w319:string)  [unwired: 2 out]
          n107 = Decimal String To Number(string=w324) -> (number=w338:i32)  [unwired: 2 in, 1 out]
          n108 = Build Array(w340, w339) -> (w336:i16[])
          n109 = Decrement(x=w338) -> (x-1=w337:i32)
          n110 = Fract/Exp String To Number(string=w345) -> (number=w346:dbl)  [unwired: 3 in, 1 out]
          n111 = Index Array(array=w336, index=w337) -> (element=w335:i16)
          n112 = Decrement(x=w335) -> (x-1=w332:i16)
          n113 = Multiply(x=2, y=w332) -> (x*y=w333:i32)
          n114 = Add(x=1, y=w333) -> (x+y=w330:i32)
          n115 = call "Set DAC Offset.vi"("error in (no error)"=w350, "DAC Offset (0)"=w346, "Axis (1)"=w330, "VISA resource name"=w351) -> ("error out"=w328:errorcluster, "VISA resource name out"=w329:refnum<visa-resource-name>)  [unwired: 2 in]
          n116 = call "createCommandListForCommandCase.vi"("immediate Check (only once)"=TRUE, "setvalue"=w345) -> ("new commands"=w326:string)  [unwired: 9 in]
          n117 = Concatenate Strings("\nsetPower.Axis ", w324) -> (w321:string)
          n118 = Concatenate Strings(w321, ">>off ") -> (w316:string)
          n119 = Concatenate Strings("\nget" ("string"), w319) -> (w314:string)
          n120 = Concatenate Strings(w321, ">>on ") -> (w315:string)
          n121 = Concatenate Strings(w316, "\n", w315, w314) -> (w313:string)
          n122 = Bundle By Name(cluster=w343, "Settings"=w327, "Connection"=w329) -> (w342:refnum<class "Tapedrive_ESP301.lvclass">)
          n123 = Concatenate Strings(w326, w313) -> (w325:string)
        }
        frame "setMoveAcceleration", "setMoveDecceleration", "setMoveVelocity", "setTensionAcceleration", "setTensionDecceleration", "setTensionVelocity" {
          n124 = call "reBuildJoindCommand.vi"("number of group elements (0)"=1, "Args"=w372, "Command 2"=w365) -> ("Arg"=w370:string, "Command"=w364:string)
          n125 = Unbundle By Name(w368) -> ("Settings"=w357:T5)
          n126 = Fract/Exp String To Number(string=w370) -> (number=w356:dbl)  [unwired: 3 in, 1 out]
          n127 = call "createCommandListForCommandCase.vi"("immediate Check (only once)"=TRUE, "setvalue"=w370, "command"=w364) -> ("new commands"=w362:string)  [unwired: 8 in]
          n128 = call "CheckIfSetCommand.vi"("Command"=w364) -> ("variable"=w358:string)  [unwired: 2 out]
          n129 = Concatenate Strings(w358, ".Value" ("string")) -> (w353:string)
          n130 = call "CompressAndUpdate(Numeric).vi"("force CVT update (false)"=TRUE, "error in"=w361, "Numeric"=w356, "command or variable name"=w364) -> ("error out"=w355:errorcluster)  [unwired: 7 in]
          n131 = call "Set Cluster Element by Name__ogtk_TS.vi"("error in (no error)"=w355, "Element Name (\"\": New Element Data Name)"=w353, "New Element Value"=w356, "Cluster"=w357) -> ("error out"=w352:errorcluster, "VCluster out"=w354:variant)  [unwired: 5 in, 1 out]
          n132 = Variant To Data(error in=w352, type=w357, Variant=w354) -> (data=w367:T5, error out=w360:errorcluster)
          n133 = Bundle By Name(cluster=w368, "Settings"=w367) -> (w366:refnum<class "Tapedrive_ESP301.lvclass">)
        }
        frame "getAcceleration", "getAccelerationFFG", "getDACoffset", "getDecceleration", "getMaxAcceleration", "getMaxVelocity", "getVelocity", "getVelocityFFG" {
          n134 = Unbundle By Name(w398) -> ("Settings"=w396:T5, "forwardaxis"=w384:i16, "backwardaxis"=w383:i16)
          n135 = call "reBuildJoindCommand.vi"("number of group elements (0)"=1, "Args"=w405, "Command 2"=w390) -> ("Arg"=w401:string, "Command"=w374:string)
          n136 = call "getSeperator.vi"("Channel Seperator (\"\")"=w403, "Command"=w374) -> ("Channel"=w402:string)  [unwired: 8 in, 1 out]
          n137 = Decimal String To Number(string=w402) -> (number=w382:i32)  [unwired: 2 in, 1 out]
          n138 = Decrement(x=w382) -> (x-1=w381:i32)
          n139 = Build Array(w384, w383) -> (w380:i16[])
          n140 = Index Array(array=w380, index=w381) -> (element=w379:i16)
          n141 = call "CheckIfSetCommand.vi"("Command"=w390) -> ("variable"=w389:string)  [unwired: 2 out]
          n142 = case shown="\"DACoffset\"" w389 {
            tunnel: w391 -> [w407 w412 w419 w426 w430 w436 w442 w449]
            tunnel: w392 -> [w406 w413 w418 w425 w432 w437 w443 w453]
            tunnel: w379 -> [w410 w417 w420 w424 w431 w439 w444 w454]
            tunnel: [w408 w416 w421 w427 w433 w438 w445 w452] -> w387
            tunnel: [w409 w415 w422 w428 w435 w440 w446 w451] -> w386
            tunnel: [w411 w414 w423 w429 w434 w441 w447 w450] -> w393
            frame "Velocity", Default {
              n143 = call "Get Velocity.vi"("error in (no error)"=w406, "Axis (1)"=w410, "VISA resource name"=w407) -> ("error out"=w408:errorcluster, "Velocity (units/s)"=w409:dbl, "VISA resource name out"=w411:refnum<visa-resource-name>)  [unwired: 2 in]
            }
            frame "Acceleration" {
              n144 = call "Get Acceleration.vi"("error in (no error)"=w413, "Axis (1)"=w417, "VISA resource name"=w412) -> ("error out"=w416:errorcluster, "Acceleration (units/s²)"=w415:dbl, "VISA resource name out"=w414:refnum<visa-resource-name>)  [unwired: 2 in]
            }
            frame "Decceleration" {
              n145 = call "Get Deceleration.vi"("error in (no error)"=w418, "Axis (1)"=w420, "VISA resource name"=w419) -> ("error out"=w421:errorcluster, "Deceleration (units/s²)"=w422:dbl, "VISA resource name out"=w423:refnum<visa-resource-name>)  [unwired: 2 in]
            }
            frame "MaxVelocity" {
              n146 = call "Get Maximum Velocity.vi"("error in (no error)"=w425, "Axis (1)"=w424, "VISA resource name"=w426) -> ("error out"=w427:errorcluster, "Maximum Velocity (units/s)"=w428:dbl, "VISA resource name out"=w429:refnum<visa-resource-name>)  [unwired: 2 in]
            }
            frame "MaxAcceleration" {
              n147 = call "Get Maximum Acceleration and Deceleration.vi"("error in (no error)"=w432, "Axis (1)"=w431, "VISA resource name"=w430) -> ("error out"=w433:errorcluster, "Acceleration (units/s²)"=w435:dbl, "VISA resource name out"=w434:refnum<visa-resource-name>)  [unwired: 2 in]
            }
            frame "VelocityFFG" {
              n148 = call "Get Velocity Feed-Forward Gain.vi"("error in (no error)"=w437, "Axis (1)"=w439, "VISA resource name"=w436) -> ("error out"=w438:errorcluster, "Gain"=w440:dbl, "VISA resource name out"=w441:refnum<visa-resource-name>)  [unwired: 2 in]
            }
            frame "AccelerationFFG" {
              n149 = call "Get Acceleration Feed-Forward Gain.vi"("error in (no error)"=w443, "Axis (1)"=w444, "VISA resource name"=w442) -> ("error out"=w445:errorcluster, "Gain"=w446:dbl, "VISA resource name out"=w447:refnum<visa-resource-name>)  [unwired: 2 in]
            }
            frame "DACoffset" {
              n150 = Decrement(x=w454) -> (x-1=w456:i16)
              n151 = Multiply(x=2, y=w456) -> (x*y=w457:i32)
              n152 = Add(x=1, y=w457) -> (x+y=w448:i32)
              n153 = call "Get DAC Offset.vi"("error in (no error)"=w453, "Axis (1)"=w448, "VISA resource name"=w449) -> ("error out"=w452:errorcluster, "DAC Offset"=w451:dbl, "VISA resource name out"=w450:refnum<visa-resource-name>)  [unwired: 2 in]
            }
          }
          n154 = call "createCommandListForCommandCase.vi"("immediate Check (only once)"=TRUE, "setvalue"=w401, "command"=w374) -> ("new commands"=w399:string)  [unwired: 8 in]
          n155 = call "CheckIfSetCommand.vi"("Command"=w374) -> ("variable"=w373:string)  [unwired: 2 out]
          n156 = call "CompressAndUpdate(Numeric).vi"("force CVT update (false)"=TRUE, "error in"=w387, "Numeric"=w386, "command or variable name"=w373) -> ("error out"=w375:errorcluster)  [unwired: 7 in]
          n157 = Concatenate Strings(w373, ".Value" ("string")) -> (w377:string)
          n158 = call "Set Cluster Element by Name__ogtk_TS.vi"("error in (no error)"=w375, "Element Name (\"\": New Element Data Name)"=w377, "New Element Value"=w386, "Cluster"=w396) -> ("error out"=w376:errorcluster, "VCluster out"=w397:variant)  [unwired: 5 in, 1 out]
          n159 = Variant To Data(error in=w376, type=w396, Variant=w397) -> (data=w395:T5, error out=w388:errorcluster)
          n160 = Bundle By Name(cluster=w398, "Settings"=w395, "Connection"=w393) -> (w394:refnum<class "Tapedrive_ESP301.lvclass">)
        }
        frame "setPower" {
          n161 = call "reBuildJoindCommand.vi"("number of group elements (0)"=1, "Args"=w483, "Command 2"=w497) -> ("Arg"=w493:string, "Command"=w474:string)
          "Command" <- w474
          n162 = Unbundle By Name(w490) -> ("Settings"=w467:T5, "forwardaxis"=w464:i16, "backwardaxis"=w463:i16)
          n163 = call "getSeperator.vi"("Channel Seperator (\"\")"=w495, "Command"=w474) -> ("Channel"=w494:string)  [unwired: 8 in, 1 out]
          n164 = Decimal String To Number(string=w494) -> (number=w460:i32)  [unwired: 2 in, 1 out]
          n165 = Index Array(array=w483, index=0) -> (element=w484:string)
          n166 = Decrement(x=w460) -> (x-1=w459:i32)
          n167 = case shown="\"on\"" w484 {
            tunnel: [FALSE TRUE] -> w476
            frame "off", Default {
            }
            frame "on" {
            }
          }
          n168 = Build Array(w464, w463) -> (w461:i16[])
          n169 = Index Array(array=w461, index=w459) -> (element=w462:i16)
          n170 = call "Enable Disable Motor.vi"("error in (no error)"=w486, "Action (OFF)"=w476, "Axis (1)"=w462, "VISA resource name"=w487) -> ("error out"=w481:errorcluster, "VISA resource name out"=w482:refnum<visa-resource-name>)  [unwired: 2 in]
          n171 = call "Get Motor Power Status.vi"("error in (no error)"=w481, "Wait before read (0ms)"=u32 100, "Axis (1)"=w462, "VISA resource name"=w482) -> ("error out"=w475:errorcluster, "Power Status"=w477:bool, "VISA resource name out"=w480:refnum<visa-resource-name>)  [unwired: 1 in]
          n172 = call "createCommandListForCommandCase.vi"("immediate Check (only once)"=TRUE, "setvalue"=w493, "command"=w474) -> ("new commands"=w491:string)  [unwired: 8 in]
          n173 = Select(t=OnOffTypeDef."on" ("Settings.inmotion"), s=w477, f=OnOffTypeDef."off" ("Settings.inmotion")) -> (s? t:f=w465:T2)
          n174 = call "CheckIfSetCommand.vi"("Command"=w474) -> ("variable"=w466:string)  [unwired: 2 out]
          n175 = call "CompressAndUpdate(Enum).vi"("force CVT update (false)"=TRUE, "error in"=w475, "enum variant"=w465, "command or variable name"=w474) -> ("error out"=w470:errorcluster)  [unwired: 7 in]
          n176 = call "Set Cluster Element by Name__ogtk_TS.vi"("error in (no error)"=w470, "Element Name (\"\": New Element Data Name)"=w466, "New Element Value"=w465, "Cluster"=w467) -> ("error out"=w469:errorcluster, "VCluster out"=w468:variant)  [unwired: 5 in, 1 out]
          n177 = Variant To Data(error in=w469, type=w467, Variant=w468) -> (data=w489:T5, error out=w471:errorcluster)
          n178 = Bundle By Name(cluster=w490, "Settings"=w489, "Connection"=w480) -> (w488:refnum<class "Tapedrive_ESP301.lvclass">)
        }
        frame "getPower" {
          n179 = call "reBuildJoindCommand.vi"("number of group elements (0)"=1, "Args"=w517, "Command 2"=w527) -> ("Arg"=w523:string, "Command"=w508:string)
          n180 = call "getSeperator.vi"("Channel Seperator (\"\")"=w525, "Command"=w508) -> ("Channel"=w524:string)  [unwired: 8 in, 1 out]
          n181 = Decimal String To Number(string=w524) -> (number=w516:i32)  [unwired: 2 in, 1 out]
          n182 = call "Get Motor Power Status.vi"("error in (no error)"=w510, "Axis (1)"=w516, "VISA resource name"=w511) -> ("error out"=w509:errorcluster, "Power Status"=w512:bool, "VISA resource name out"=w515:refnum<visa-resource-name>)  [unwired: 2 in]
          n183 = Unbundle By Name(w520) -> ("Settings"=w501:T5)
          n184 = Select(t=OnOffTypeDef."on" ("Settings.inmotion"), s=w512, f=OnOffTypeDef."off" ("Settings.inmotion")) -> (s? t:f=w502:T2)
          n185 = call "createCommandListForCommandCase.vi"("immediate Check (only once)"=TRUE, "setvalue"=w523, "command"=w508) -> ("new commands"=w521:string)  [unwired: 8 in]
          n186 = call "CheckIfSetCommand.vi"("Command"=w508) -> ("variable"=w500:string)  [unwired: 2 out]
          n187 = call "CompressAndUpdate(Enum).vi"("force CVT update (false)"=TRUE, "error in"=w509, "enum variant"=w502, "command or variable name"=w500) -> ("error out"=w504:errorcluster)  [unwired: 7 in]
          n188 = call "Set Cluster Element by Name__ogtk_TS.vi"("error in (no error)"=w504, "Element Name (\"\": New Element Data Name)"=w500, "New Element Value"=w502, "Cluster"=w501) -> ("error out"=w505:errorcluster, "VCluster out"=w503:variant)  [unwired: 5 in, 1 out]
          n189 = Variant To Data(error in=w505, type=w501, Variant=w503) -> (data=w519:T5, error out=w506:errorcluster)
          n190 = Bundle By Name(cluster=w520, "Settings"=w519, "Connection"=w515) -> (w518:refnum<class "Tapedrive_ESP301.lvclass">)
        }
        frame "putMasterSlave" {
          n191 = Unbundle By Name(w545) -> ("Connection"=w547:refnum<visa-resource-name>, "forwardaxis"=w549:i16, "backwardaxis"=w548:i16)
          n192 = Index Array(array=w555, index=0) -> (element=w554:string)
          n193 = case shown="\"Forward\", Default" w554 {
            tunnel: w549 -> [w558 w562]
            tunnel: w548 -> [w559 w561]
            tunnel: [w559 w562] -> w528
            tunnel: [w558 w561] -> w529
            tunnel: [w557 w560] -> w536
            frame "Backward" {
              w557 = Direction."Backward"  # Direction
            }
            frame "Forward", Default {
              w560 = Direction."Forward"  # Direction
            }
          }
          n194 = call "Define Master Slave Relationship.vi"("error in (no error)"=w546, "Master Axis"=w528, "Slave Axis"=w529, "VISA resource name"=w547) -> ("error out"=w551:errorcluster, "VISA resource name out"=w550:refnum<visa-resource-name>)  [unwired: 2 in]
          n195 = call "Set Trajectory Mode.vi"("Trajectory Mode"=T4."Slave to master's desired position (trajectory)", "error in (no error)"=w551, "Axis (1)"=w529, "VISA resource name"=w550) -> ("error out"=w553:errorcluster, "VISA resource name out"=w552:refnum<visa-resource-name>)  [unwired: 3 in]
          n196 = call "Set Trajectory Mode.vi"("Trajectory Mode"=T4."Trapezoidal Mode", "error in (no error)"=w553, "Axis (1)"=w528, "VISA resource name"=w552) -> ("error out"=w543:errorcluster, "VISA resource name out"=w541:refnum<visa-resource-name>)  [unwired: 3 in]
          n197 = call "Get Master-Slave Relationship.vi"("error in (no error)"=w543, "Slave Axis"=w529, "VISA resource name"=w541) -> ("error out"=w533:errorcluster, "Master Axis"=w538:i32, "VISA resource name out"=w542:refnum<visa-resource-name>)  [unwired: 2 in]
          n198 = Equal?(x=w528, y=w538) -> (x = y?=w537:bool)
          n199 = Select(t=w536, s=w537, f=Direction."Undefined") -> (s? t:f=w534:T3)
          n200 = Bundle By Name(cluster=w545, "Direction"=w534, "Connection"=w542) -> (w544:refnum<class "Tapedrive_ESP301.lvclass">)
          n201 = call "CompressAndUpdate(Enum).vi"("force CVT update (false)"=TRUE, "error in"=w533, "enum variant"=w534, "command or variable name"="Direction") -> ("error out"=w532:errorcluster)  [unwired: 7 in]
        }
        frame "putReleaseSlaving" {
          w567 = T4."Trapezoidal Mode" ("Trajectory Mode")
          n202 = Unbundle By Name(w573) -> ("forwardaxis"=w576:i16, "backwardaxis"=w575:i16)
          n203 = call "Set Trajectory Mode.vi"("Trajectory Mode"=w567, "error in (no error)"=w574, "Axis (1)"=w575, "VISA resource name"=w577) -> ("error out"=w569:errorcluster, "VISA resource name out"=w568:refnum<visa-resource-name>)  [unwired: 3 in]
          n204 = call "Set Trajectory Mode.vi"("Trajectory Mode"=w567, "error in (no error)"=w569, "Axis (1)"=w576, "VISA resource name"=w568) -> ("error out"=w563:errorcluster, "VISA resource name out"=w564:refnum<visa-resource-name>)  [unwired: 3 in]
          n205 = call "Define Master Slave Relationship.vi"("error in (no error)"=w563, "Master Axis"=w575, "Slave Axis"=w575, "VISA resource name"=w564) -> ("error out"=w566:errorcluster, "VISA resource name out"=w565:refnum<visa-resource-name>)  [unwired: 2 in]
          n206 = call "Define Master Slave Relationship.vi"("error in (no error)"=w566, "Master Axis"=w576, "Slave Axis"=w576, "VISA resource name"=w565) -> ("error out"=w570:errorcluster, "VISA resource name out"=w572:refnum<visa-resource-name>)  [unwired: 2 in]
          n207 = Bundle By Name(cluster=w573, "Connection"=w572) -> (w571:refnum<class "Tapedrive_ESP301.lvclass">)
        }
        frame "Wait" {
          n208 = Index Array(array=w580) -> (element=w579:string)  [unwired: 1 in]
          n209 = Fract/Exp String To Number(string=w579) -> (number=w578:dbl)  [unwired: 3 in, 1 out]
          n210 = Wait (ms)(milliseconds to wait=w578) -> ()  [unwired: 1 out]
        }
        frame "putStep" {
          n211 = Unbundle By Name(w589) -> ("forwardaxis"=w584:i16, "Velocity"=w605:T6, "Acceleration"=w604:T6, "Decceleration"=w603:T6, "MoveVelocity"=w602:T6, "MoveAcceleration"=w601:T6, "MoveDecceleration"=w600:T6, "Tension"=w590:T2)  [unwired: 1 out]
          n212 = Build Array(w602, w601, w600) -> (w598:T7)
          n213 = Build Array(w605, w604, w603) -> (w599:T7)
          n214 = case shown="\"on\"" w590 {
            tunnel: w594 -> [w608 w611]
            tunnel: [w608 w610] -> w593
            tunnel: w592 -> [w607 w614]
            tunnel: w584 -> [_ w613]
            tunnel: [w607 w609] -> w591
            frame "off", Default {
            }
            frame "on" {
              n215 = call "Stop Motion.vi"("error in (no error)"=w611, "Stop all axes (F)"=TRUE, "Axis (1)"=w613, "VISA resource name"=w614) -> ("error out"=w610:errorcluster, "VISA resource name out"=w609:refnum<visa-resource-name>)  [unwired: 2 in]
            }
          }
          n216 = call "set_Mode.vi"("Array"=w598, "Array 3"=string[] ["Velocity", "Acceleration", "Decceleration"], "Array 2"=w599) -> ("settings needed"=w597:bool, "spreadsheet string"=w596:string)  [unwired: 7 in]
          n217 = case shown="False" w597 {
            tunnel: w596 -> [_ w642]
            tunnel: ["" w640] -> w595
            tunnel: w593 -> [w629 w644]
            tunnel: w591 -> [w628 w643]
            tunnel: w589 -> [w639 w645]
            tunnel: [w638 w645] -> w587
            tunnel: [w634 w644] -> w588
            tunnel: [w633 w643] -> w585
            tunnel: [TRUE ("Wait for Step") FALSE ("Wait for Step")] -> w583
            frame False {
              n218 = Unbundle By Name(w639) -> ("Value"=w636:dbl, "Value"=w637:dbl, "forwardaxis"=w632:i16, "backwardaxis"=w630:i16, "Direction"=w635:T3)
              n219 = call "direction_axis.vi"("Direction"=w635, "backwardaxis"=w630, "forwardaxis"=w632) -> ("Slave"=w618:i16, "Master"=w631:i16)  [unwired: 7 in]
              n220 = call "Set Master-Slave Reduction Ratio.vi"("error in (no error)"=w629, "Reduction Ratio (0)"=0.0, "Axis (1)"=w618, "VISA resource name"=w628) -> ("error out"=w626:errorcluster, "VISA resource name out"=w625:refnum<visa-resource-name>)  [unwired: 2 in]
              n221 = call "Get Master-Slave Reduction Ratio.vi"("error in (no error)"=w626, "Axis (1)"=w618, "VISA resource name"=w625) -> ("error out"=w622:errorcluster, "Reduction Ratio"=w619:dbl, "VISA resource name out"=w624:refnum<visa-resource-name>)  [unwired: 2 in]
              n222 = call "CompressAndUpdate(Numeric).vi"("force CVT update (false)"=TRUE, "error in"=w622, "Numeric"=w619, "command or variable name"="RedRatio") -> ("error out"=w621:errorcluster)  [unwired: 7 in]
              n223 = call "Move Relative.vi"("error in (no error)"=w621, "Position (0 units)"=w636, "Axis (1)"=w631, "VISA resource name"=w624) -> ("error out"=w634:errorcluster, "VISA resource name out"=w633:refnum<visa-resource-name>)  [unwired: 2 in]
              n224 = Tick Count (ms)() -> (millisecond timer value=w615:u32)
              n225 = Bundle By Name(cluster=w639, "startpos"=w637, "startTime"=w615) -> (w638:refnum<class "Tapedrive_ESP301.lvclass">)
            }
            frame True {
              n226 = disable-structure shown="Enabled" {
                disable-tunnel: w642 -> [w649 w650]
                disable-tunnel: [w646 w650] -> w640
                frame Enabled {
                  n227 = Concatenate Strings(w649, "\n", "putStep") -> (w646:string)
                }
                frame Disabled {
                }
              }
            }
          }
          n228 = Bundle By Name(cluster=w587, "Connection"=w585, "Moving?"=w583) -> (w586:refnum<class "Tapedrive_ESP301.lvclass">)
        }
        frame "setReductionRatio" {
          n229 = Unbundle By Name(w661) -> ("forwardaxis"=w668:i16, "backwardaxis"=w667:i16, "Direction"=w666:T3)
          n230 = Index Array(array=w664) -> (element=w663:string)  [unwired: 1 in]
          n231 = Fract/Exp String To Number(string=w663) -> (number=w662:dbl)  [unwired: 3 in, 1 out]
          n232 = call "direction_axis.vi"("Direction"=w666, "backwardaxis"=w667, "forwardaxis"=w668) -> ("Slave"=w657:i16)  [unwired: 7 in, 1 out]
          n233 = call "Set Master-Slave Reduction Ratio.vi"("error in (no error)"=w665, "Reduction Ratio (0)"=w662, "Axis (1)"=w657, "VISA resource name"=w669) -> ("error out"=w658:errorcluster, "VISA resource name out"=w659:refnum<visa-resource-name>)  [unwired: 2 in]
          n234 = call "Get Master-Slave Reduction Ratio.vi"("error in (no error)"=w658, "Axis (1)"=w657, "VISA resource name"=w659) -> ("error out"=w655:errorcluster, "Reduction Ratio"=w651:dbl, "VISA resource name out"=w656:refnum<visa-resource-name>)  [unwired: 2 in]
          n235 = call "CompressAndUpdate(Numeric).vi"("force CVT update (false)"=TRUE, "error in"=w655, "Numeric"=w651, "command or variable name"=w653) -> ("error out"=w654:errorcluster)  [unwired: 7 in]
          n236 = Bundle By Name(cluster=w661, "Connection"=w656, "Value"=w651) -> (w660:refnum<class "Tapedrive_ESP301.lvclass">)
        }
        frame "putTension" {
          n237 = Unbundle By Name(w675) -> ("forwardaxis"=w670:i16, "Velocity"=w691:T6, "Acceleration"=w690:T6, "Decceleration"=w689:T6, "TensionVelocity"=w688:T6, "TensionAcceleration"=w687:T6, "TensionDecceleration"=w686:T6, "Tension"=w676:T2)  [unwired: 2 out]
          n238 = Build Array(w688, w687, w686) -> (w684:T7)
          n239 = Build Array(w691, w690, w689) -> (w685:T7)
          n240 = case shown="\"on\"" w676 {
            tunnel: w680 -> [w694 w697]
            tunnel: [w694 w696] -> w679
            tunnel: w678 -> [w693 w700]
            tunnel: w670 -> [_ w699]
            tunnel: [w693 w695] -> w677
            frame "off", Default {
            }
            frame "on" {
              n241 = call "Stop Motion.vi"("error in (no error)"=w697, "Stop all axes (F)"=TRUE, "Axis (1)"=w699, "VISA resource name"=w700) -> ("error out"=w696:errorcluster, "VISA resource name out"=w695:refnum<visa-resource-name>)  [unwired: 2 in]
            }
          }
          n242 = call "set_Mode.vi"("Array"=w684, "Array 3"=string[] ["Velocity", "Acceleration", "Decceleration"], "Array 2"=w685) -> ("settings needed"=w683:bool, "spreadsheet string"=w682:string)  [unwired: 7 in]
          n243 = case shown="False" w683 {
            tunnel: w682 -> [_ w731]
            tunnel: ["" w730] -> w681
            tunnel: w679 -> [w715 w733]
            tunnel: w677 -> [w714 w732]
            tunnel: w675 -> [w725 w734]
            tunnel: [w724 w734] -> w673
            tunnel: [w702 w733] -> w674
            tunnel: [w720 w732] -> w671
            frame False {
              n244 = Unbundle By Name(w725) -> ("Value"=w722:dbl, "Value"=w723:dbl, "forwardaxis"=w716:i16, "backwardaxis"=w717:i16, "Direction"=w721:T3, "Value"=w701:dbl)
              n245 = call "direction_axis.vi"("Direction"=w721, "backwardaxis"=w717, "forwardaxis"=w716) -> ("Slave"=w704:i16, "Master"=w718:i16)  [unwired: 7 in]
              n246 = call "Set Master-Slave Reduction Ratio.vi"("error in (no error)"=w715, "Reduction Ratio (0)"=1.0, "Axis (1)"=w704, "VISA resource name"=w714) -> ("error out"=w710:errorcluster, "VISA resource name out"=w712:refnum<visa-resource-name>)  [unwired: 2 in]
              n247 = call "Get Master-Slave Reduction Ratio.vi"("error in (no error)"=w710, "Axis (1)"=w704, "VISA resource name"=w712) -> ("error out"=w709:errorcluster, "Reduction Ratio"=w707:dbl, "VISA resource name out"=w711:refnum<visa-resource-name>)  [unwired: 2 in]
              n248 = call "CompressAndUpdate(Numeric).vi"("force CVT update (false)"=TRUE, "error in"=w709, "Numeric"=w707, "command or variable name"="RedRatio") -> ("error out"=w708:errorcluster)  [unwired: 7 in]
              n249 = Bundle By Name(cluster=w725, "startpos"=w723) -> (w724:refnum<class "Tapedrive_ESP301.lvclass">)
              n250 = call "Move Relative.vi"("error in (no error)"=w708, "Position (0 units)"=w722, "Axis (1)"=w718, "VISA resource name"=w711) -> ("error out"=w703:errorcluster, "VISA resource name out"=w720:refnum<visa-resource-name>)  [unwired: 2 in]
              n251 = flat-sequence {
                tunnel: w703 -> [w727]
                tunnel: [w727] -> w702
                tunnel: w701 -> [w726]
                frame #0 {
                  n252 = Wait (ms)(milliseconds to wait=w726) -> ()  [unwired: 1 out]
                }
              }
            }
            frame True {
              n253 = Concatenate Strings(w731, "\n", "putTension") -> (w730:string)
            }
          }
          n254 = Bundle By Name(cluster=w673, "Connection"=w671) -> (w672:refnum<class "Tapedrive_ESP301.lvclass">)
        }
        frame "setDirection" {
          n255 = Unbundle By Name(w739) -> ("forwardaxis"=w744:i16, "status"=w746:T8, "Tension"=w740:T2)
          n256 = Index Array(array=w748) -> (element=w747:string)  [unwired: 1 in]
          n257 = case shown="\"Moving\"" w746 {
            tunnel: w745 -> [w754 w760]
            tunnel: w744 -> [_ w759]
            tunnel: w743 -> [w753 w757]
            tunnel: [w753 w756] -> w742
            tunnel: [w754 w755] -> w737
            frame Default {
            }
            frame "Moving" {
              n258 = call "Stop Motion.vi"("error in (no error)"=w757, "Stop all axes (F)"=TRUE, "Axis (1)"=w759, "VISA resource name"=w760) -> ("error out"=w756:errorcluster, "VISA resource name out"=w755:refnum<visa-resource-name>)  [unwired: 2 in]
            }
          }
          n259 = Concatenate Strings("putReleaseSlaving\nputMasterSlave>>", w747) -> (w736:string)
          n260 = case shown="\"on\"" w740 {
            tunnel: w736 -> [w749 w752]
            tunnel: [w749 w750] -> w735
            frame "off", Default {
            }
            frame "on" {
              n261 = Concatenate Strings(w752, "putTension" ("string")) -> (w750:string)
            }
          }
          n262 = Bundle By Name(cluster=w739, "Connection"=w737) -> (w738:refnum<class "Tapedrive_ESP301.lvclass">)
        }
        frame "Abort" {
          n263 = Index Array(array=w762) -> (element=w761:string)  [unwired: 1 in]
          n264 = case shown="\"ClearQueue\"" w761 {
            tunnel: [w768 w791] -> w767
            tunnel: w766 -> [w768 w790]
            tunnel: w765 -> [_ w789]
            tunnel: w764 -> [w769 w788]
            tunnel: [w769 w774] -> w763
            frame "ClearQueue" {
            }
            frame Default {
              w773 = TRUE ("force CVT update (false)")
              w777 = FALSE ("Action (OFF)")
              n265 = Unbundle By Name(w790) -> ("forwardaxis"=w782:i16, "backwardaxis"=w781:i16)
              n266 = call "Stop Motion.vi"("error in (no error)"=w788, "Stop all axes (F)"=TRUE, "Axis (1)"=w782, "VISA resource name"=w789) -> ("error out"=w785:errorcluster, "VISA resource name out"=w786:refnum<visa-resource-name>)  [unwired: 2 in]
              n267 = call "Enable Disable Motor.vi"("error in (no error)"=w785, "Action (OFF)"=w777, "Axis (1)"=w782, "VISA resource name"=w786) -> ("error out"=w784:errorcluster, "VISA resource name out"=w780:refnum<visa-resource-name>)  [unwired: 2 in]
              n268 = call "Enable Disable Motor.vi"("error in (no error)"=w784, "Action (OFF)"=w777, "Axis (1)"=w781, "VISA resource name"=w780) -> ("error out"=w776:errorcluster, "VISA resource name out"=w783:refnum<visa-resource-name>)  [unwired: 2 in]
              n269 = Bundle By Name(cluster=w790, "Connection"=w783) -> (w791:refnum<class "Tapedrive_ESP301.lvclass">)
              n270 = Select(t=OnOffTypeDef."on" ("Settings.inmotion"), s=w777, f=OnOffTypeDef."off" ("Settings.inmotion")) -> (s? t:f=w772:T2)
              n271 = call "CompressAndUpdate(Enum).vi"("force CVT update (false)"=w773, "error in"=w776, "enum variant"=w772, "command or variable name"="setPower.Axis 1" ("Seperator out")) -> ("error out"=w775:errorcluster)  [unwired: 7 in]
              n272 = call "CompressAndUpdate(Enum).vi"("force CVT update (false)"=w773, "error in"=w775, "enum variant"=w772, "command or variable name"="setPower.Axis 2" ("Seperator out")) -> ("error out"=w774:errorcluster)  [unwired: 7 in]
            }
          }
        }
      }
      n273 = case shown="True" w20 {
        tunnel: w24 -> [w26 w35]
        tunnel: [w26 w34] -> w23
        tunnel: [w27 w33] -> w17
        tunnel: w22 -> [w25 w32]
        tunnel: [w25 w31] -> w21
        tunnel: w8 -> [w28 w30]
        tunnel: [w28 w29] -> w19
        tunnel: w18 -> [w27 _]
        frame False {
        }
        frame True {
          n274 = call-parent "Configure.vi"("error in (no error)"=w32, "Msg in"=w30, "BaseDriver in"=w35) -> ("error out"=w31:errorcluster, "new command"=w33:string, "Msg out"=w29:T1, "BaseDriver out"=w34:refnum<class "Tapedrive_ESP301.lvclass">)  [unwired: 5 in]
        }
      }
    }
    frame Error {
    }
  }
  "error out" <- w4
  "FakePressureController out" <- w3
  "new command" <- w1
  "Msg out" <- w2
  n275 = disable-structure shown="Disabled" {
    frame Disabled {
      (unwired) OnOffTypeDef."off" ("inmotion")
      n276 = call "Set Deceleration.vi"() -> ()  [unwired: 6 in, 2 out]
      n277 = call "Set Velocity.vi"() -> ()  [unwired: 6 in, 2 out]
      n278 = call "CheckIfSetCommand.vi"() -> ()  [unwired: 1 in, 3 out]
      n279 = call "Set Maximum Acceleration and Deceleration.vi"() -> ()  [unwired: 6 in, 2 out]
      n280 = call "Set Maximum Velocity.vi"() -> ()  [unwired: 6 in, 2 out]
      n281 = call "Get Master-Slave Velocity Update Interval.vi"() -> ()  [unwired: 5 in, 3 out]
      n282 = call "CheckIfSetCommand.vi"() -> ()  [unwired: 1 in, 3 out]
      n283 = call "Get Master-Slave Velocity Update Interval.vi"() -> ()  [unwired: 5 in, 3 out]
    }
    frame Enabled {
    }
  }
